vi "Result File.vi"(7 "File name suffix":string, 10 "File Type":string, 11 "DesignRequest":T1) -> (2 "File string":string, 3 "File path":path)   [LabVIEW 2012, in "Design Server.lvlib"]
uses:
  Design Server.lvlib
  Design Request.ctl
  Variable cluster.ctl
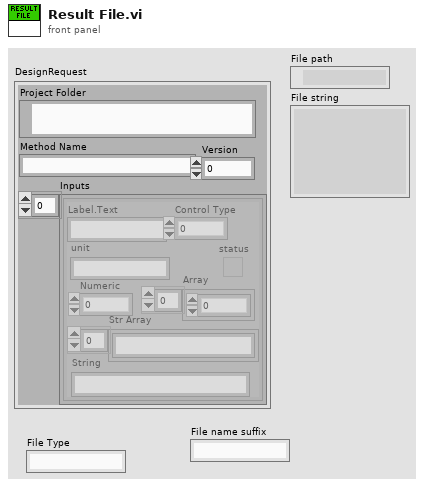
[diagram p1: front panel]
types:
  T1 = typedef "Design Server.lvlib/Design Request.ctl" = cluster{"Project Folder":path, "Method Name":string, "Inputs":T2, "Version":i32}
  T2 = typedef "Design Server.lvlib/Variable cluster.ctl" = cluster{"Label.Text":string, "Control Type":u32, "Numeric":dbl, "Array":dbl[], "status":bool, "Str Array":string[], "String":string, "unit":string}[]
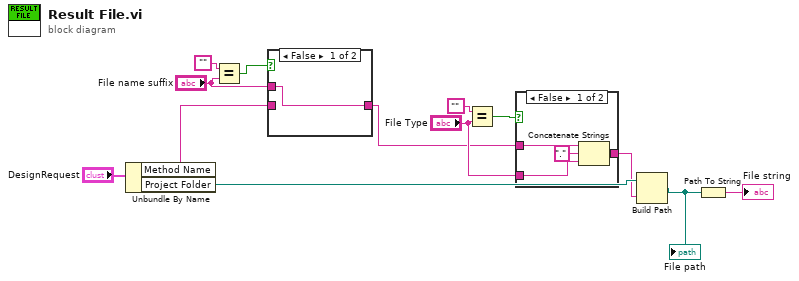
[diagram p0: block diagram]
diagram:
  n1 = Unbundle By Name("DesignRequest") -> ("Method Name"=w3:string, "Project Folder"=w12:path)
  n2 = Equal?(x="", y="File name suffix") -> (x = y?=w4:bool)
  n3 = case shown="False" w4 {
    tunnel: w3 -> [_ w15]
    tunnel: [w14 w15] -> w2
    tunnel: "File name suffix" -> [w14 _]
    frame False {
    }
    frame True {
    }
  }
  n4 = Equal?(x="", y="File Type") -> (x = y?=w7:bool)
  n5 = case shown="False" w7 {
    tunnel: "File Type" -> [w19 _]
    tunnel: [w18 w20] -> w10
    tunnel: w2 -> [w17 w20]
    frame False {
      n6 = Concatenate Strings(w17, "." ("string"), w19) -> (w18:string)
    }
    frame True {
    }
  }
  n7 = Build Path(base path=w12, name or relative path=w10) -> (appended path=w13:path)
  "File path" <- w13
  n8 = Path To String(path=w13) -> (string=→"File string":string)
